vi "Read settings.vi"(8 "error in (no error)":errorcluster) -> (0 "error out":errorcluster, 3 "Type Signal":T1={"DAQ Board Name"="DAQ_Simu1", "Analogicos Canales"=["DAQ_Simu1/ai1", "DAQ_Simu1/ai2"], "rate"=1000.0, "number of samples "=1000, "Tiempo"=100})   [LabVIEW 2020, in "Settings.lvlib"]
uses:
  Settings.lvlib
  typeSignal--cluster.ctl
  <vilib>/drjdpowell/SQLite Library/SQL Connection/Open (path).vi
  <vilib>/drjdpowell/SQLite Library/SQL Connection/Open (string).vi
  <vilib>/AdvancedString/Path To Command Line String.vi
  <vilib>/drjdpowell/SQLite Library/SQL Connection/Execute SQL (1D UTF-8).vi
  <vilib>/drjdpowell/SQLite Library/SQL Connection/Connection.lvclass
  <vilib>/drjdpowell/SQLite Library/SQLite.lvlib
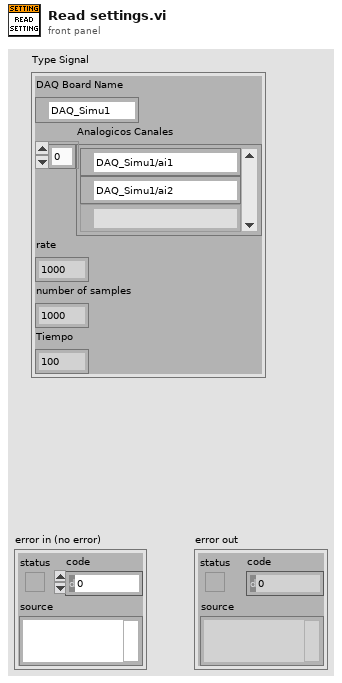
[diagram p1: front panel]
types:
  T1 = typedef "typeSignal--cluster.ctl" = cluster{"DAQ Board Name":tag, "Analogicos Canales":tag[], "rate":dbl, "number of samples ":i32, "Tiempo":i32}
  T2 = cluster{"Result Set (UTF-8)[0]":string, "Result Set (UTF-8)[1]":string, "Result Set (UTF-8)[2]":string, "Result Set (UTF-8)[3]":string, "Result Set (UTF-8)[4]":string, "Result Set (UTF-8)[5]":string, "Result Set (UTF-8)[6]":string, "Result Set (UTF-8)[7]":string, "Result Set (UTF-8)[8]":string}
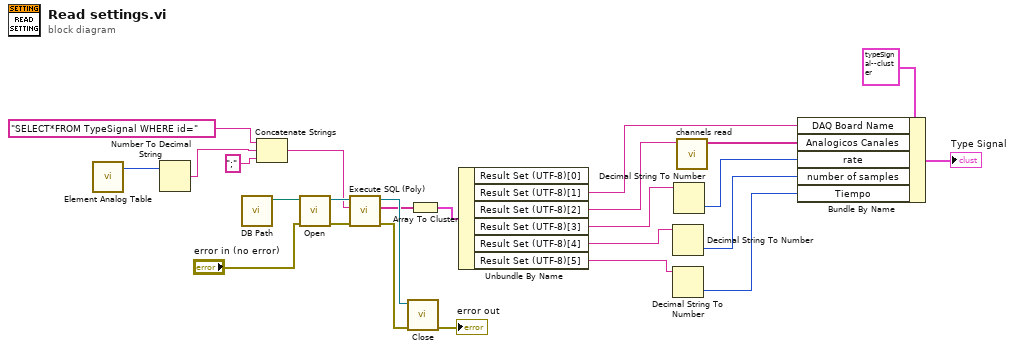
[diagram p0: block diagram]
diagram:
  n1 = call "Element Analog Table.vi"() -> ("element"=w1:i64)  [unwired: 10 in, 1 out]
  n2 = Number To Decimal String(number=w1) -> (decimal integer string=w8:string)  [unwired: 1 in]
  n3 = call "DB Path.vi"() -> ("DB path"=w16:path)  [unwired: 11 in]
  n4 = Concatenate Strings("SELECT*FROM TypeSignal WHERE id=" ("SQL"), w8, ";" ("string")) -> (w9:string)
  n5 = call-poly <vilib>:"Open.vi"("error in (no error)"="error in (no error)", "db file"=w16) -> ("error out"=w25:errorcluster, "SQLite Connection"=w24:refnum<class "Connection.lvclass">)  [unwired: 8 in]
  n6 = call-poly <vilib>:"Execute SQL (Poly).vi"("error in (no error)"=w25, "SQL"=w9, "SQLite Connection in"=w24) -> ("error out"=w22:errorcluster, "Result Set (UTF-8)"=w18:string[], "SQLite Connection"=w23:refnum<class "Connection.lvclass">)  [unwired: 5 in, 1 out]
  n7 = call-dynamic "Close.vi"("error in (no error)"=w22, "SQLite Connection in"=w23) -> ("error out"=→"error out":errorcluster)  [unwired: 9 in]
  n8 = Array To Cluster(array=w18) -> (cluster=w19:T2)
  n9 = Unbundle By Name(w19) -> ("Result Set (UTF-8)[1]"=w17:string, "Result Set (UTF-8)[2]"=w13:string, "Result Set (UTF-8)[3]"=w7:string, "Result Set (UTF-8)[4]"=w6:string, "Result Set (UTF-8)[5]"=w2:string)  [unwired: 1 out]
  n10 = Decimal String To Number(string=w6) -> (number=w4:i32)  [unwired: 2 in, 1 out]
  n11 = Decimal String To Number(string=w2) -> (number=w3:i32)  [unwired: 2 in, 1 out]
  n12 = Decimal String To Number(string=w7) -> (number=w5:i32)  [unwired: 2 in, 1 out]
  n13 = call "channels read.vi"("Result Set (UTF-8)[2]"=w13) -> ("Array"=w12:string[])  [unwired: 10 in]
  n14 = Bundle By Name(cluster=T1 {"DAQ Board Name"="DAQ_Simu1", "Analogicos Canales"=["DAQ_Simu1/ai1", "DAQ_Simu1/ai2"], "rate"=1000.0, "number of samples "=1000, "Tiempo"=100} ("Type Signal"), "DAQ Board Name"=w17, "Analogicos Canales"=w12, "rate"=w5, "number of samples"=w4, "Tiempo"=w3) -> (→"Type Signal":T1)
